vi "Timer.vi"(8 "error in (no error)":errorcluster, 10 "Set Time":dbl format="%#_13g", 11 "Timer_Enum":T1) -> (0 "error out":errorcluster, 3 "Time Out":dbl format="%#_13g")   [LabVIEW 2010]
doc: "Timer FGV for Elevator Application"
uses:
  Timer_Enum.ctl
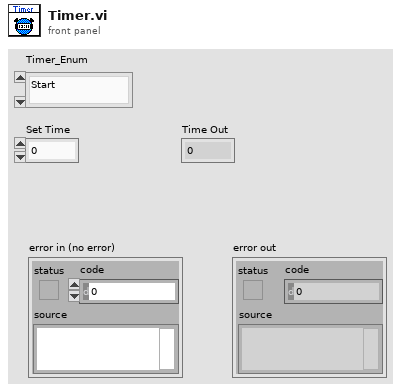
[diagram p1: front panel]
types:
  T1 = typedef "Timer_Enum.ctl" = enum16{"Start", "Read"}
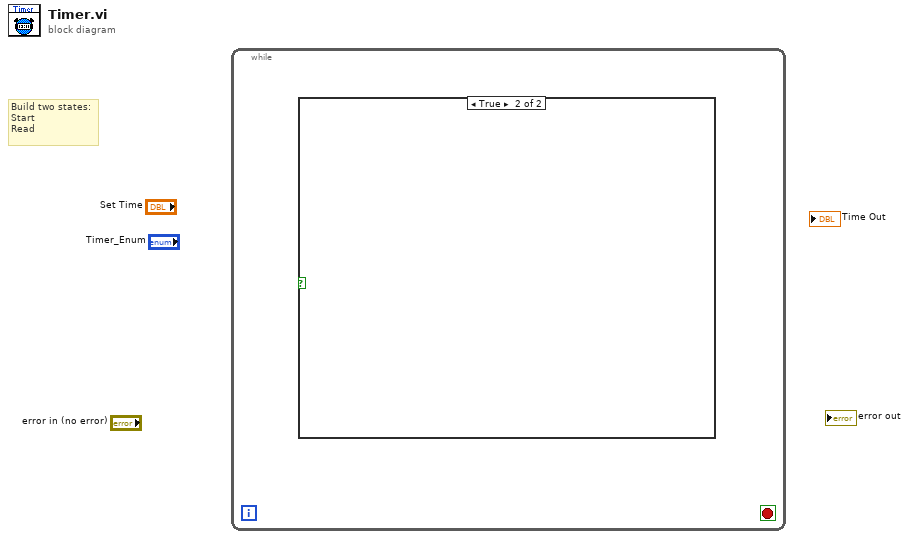
[diagram p0: block diagram]
diagram:
  # "Build two states:\nStart\nRead"
  n1 = while {
    stop <- _ stop-if-true
    n2 = case shown="True" {
      selector: _ -> [_ _]
      frame False {
      }
      frame True {
      }
    }
  }
